vi "Scrollbar einschalten.vi"(6 "Aktion":T1(ring), 11 "Fensterbereich":refnum<vi>) -> ()   [LabVIEW 2015, in "allgemeine Sub-VIs.lvlib"]
uses:
  allgemeine Sub-VIs.lvlib
  <vilib>/Utility/miscctls.llb/LVPointTypeDef.ctl
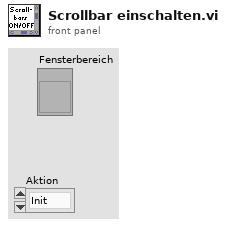
[diagram p1: front panel]
types:
  T1 = enum16{"Init", "scroll H aktiv", "scroll H inaktiv", "scroll V aktiv", "scroll V inaktiv"}
  T2 = enum16{"Always On", "Always Off", "Off While Running"}
  T3 = typedef "LVPointTypeDef.ctl" = cluster{"Horizontal":i16, "Vertical":i16}
  T4 = typedef "LVRectTypeDef.ctl" = cluster{"Left":i16, "Top":i16, "Right":i16, "Bottom":i16}
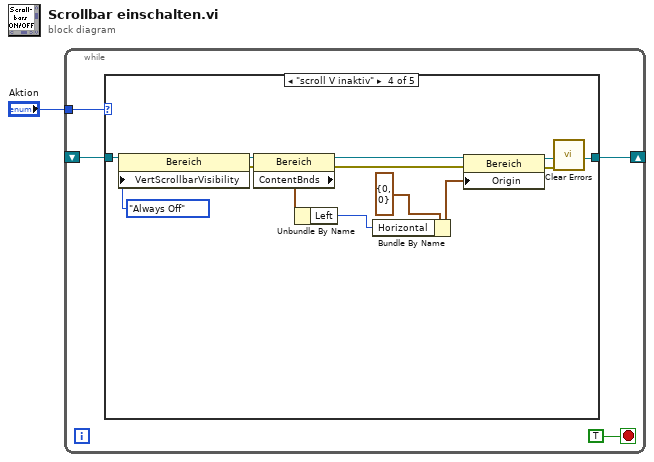
[diagram p0: block diagram]
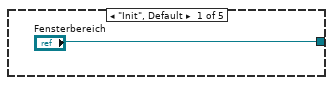
[diagram p2: hidden frame]
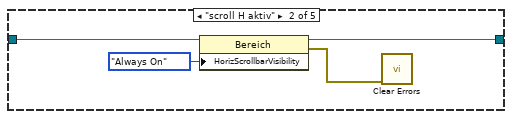
[diagram p3: hidden frame]
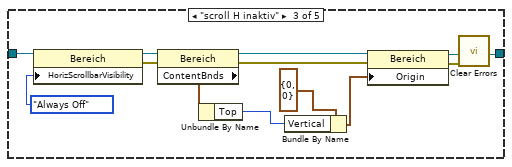
[diagram p4: hidden frame]
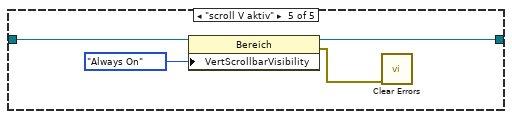
[diagram p5: hidden frame]
diagram:
  n1 = while {
    tunnel: "Aktion" -> [w4]
    shift-right: [w3] -> _
    shift-left: _ -> [w2]
    stop <- TRUE stop-if-true
    n2 = case shown="\"scroll V inaktiv\"" w4 {
      tunnel: ["Fensterbereich" w10 w12 w24 w37] -> w3
      tunnel: w2 -> [_ w7 w22 w34 w38]
      frame "Init", Default {
      }
      frame "scroll H aktiv" {
        n3 = property class="Bereich"(reference=w7, "HorizScrollbarVisibility"=T2."Always On" ("Sichtbarkeit der horizontalen Bildlaufleiste")) -> (reference out=w10:refnum<vi>, error out=w9:errorcluster)  [unwired: 1 in]
        n4 = call <vilib>:"Clear Errors.vi"("error in (no error)"=w9) -> ()  [unwired: 5 in, 2 out]
      }
      frame "scroll H inaktiv" {
        n5 = property class="Bereich"(reference=w22, "HorizScrollbarVisibility"=T2."Always Off" ("Sichtbarkeit der horizontalen Bildlaufleiste")) -> (reference out=w20:refnum<vi>, error out=w19:errorcluster)  [unwired: 1 in]
        n6 = property class="Bereich"(reference=w20, error in=w19) -> (reference out=w16:refnum<vi>, error out=w17:errorcluster, "ContentBnds"=w18:T4)
        n7 = Unbundle By Name(w18) -> ("Top"=w14:i16)
        n8 = Bundle By Name(cluster=T3 {"Horizontal"=0, "Vertical"=0} ("Ursprung"), "Vertical"=w14) -> (w13:T3)
        n9 = property class="Bereich"(reference=w16, error in=w17, "Origin"=w13) -> (reference out=w12:refnum<vi>, error out=w11:errorcluster)
        n10 = call <vilib>:"Clear Errors.vi"("error in (no error)"=w11) -> ()  [unwired: 5 in, 2 out]
      }
      frame "scroll V inaktiv" {
        n11 = property class="Bereich"(reference=w34, "VertScrollbarVisibility"=T2."Always Off" ("Sichtbarkeit der horizontalen Bildlaufleiste")) -> (reference out=w32:refnum<vi>, error out=w31:errorcluster)  [unwired: 1 in]
        n12 = property class="Bereich"(reference=w32, error in=w31) -> (reference out=w28:refnum<vi>, error out=w29:errorcluster, "ContentBnds"=w30:T4)
        n13 = Unbundle By Name(w30) -> ("Left"=w26:i16)
        n14 = Bundle By Name(cluster=T3 {"Horizontal"=0, "Vertical"=0} ("Ursprung"), "Horizontal"=w26) -> (w25:T3)
        n15 = property class="Bereich"(reference=w28, error in=w29, "Origin"=w25) -> (reference out=w24:refnum<vi>, error out=w23:errorcluster)
        n16 = call <vilib>:"Clear Errors.vi"("error in (no error)"=w23) -> ()  [unwired: 5 in, 2 out]
      }
      frame "scroll V aktiv" {
        n17 = property class="Bereich"(reference=w38, "VertScrollbarVisibility"=T2."Always On" ("Sichtbarkeit der horizontalen Bildlaufleiste")) -> (reference out=w37:refnum<vi>, error out=w36:errorcluster)  [unwired: 1 in]
        n18 = call <vilib>:"Clear Errors.vi"("error in (no error)"=w36) -> ()  [unwired: 5 in, 2 out]
      }
    }
  }
